vi "ScanXY.vi"(11 "Scan/Meas Parameters":T1={"Pixel Dwell Time (s)"=0.0001, "Pixel Size"=200.0, "X Min (V)"=-7.5, "X Max (V)"=7.5, "Y Min (V)"=-7.5, "Y Max (V)"=7.5, "XY Factor (1/V)"=0.2}) -> (3 "XYcoordinates":dbl[][](array[numeric]))   [LabVIEW 2018]
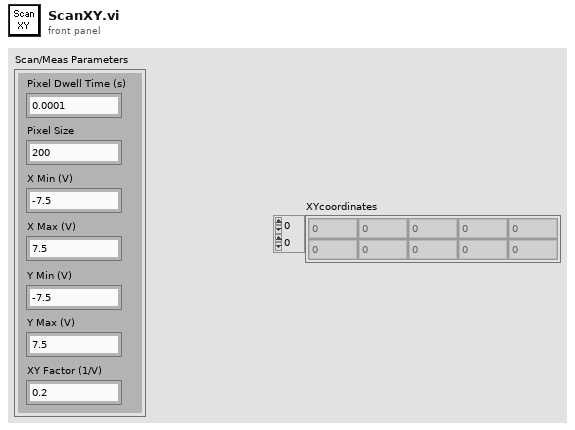
[diagram p1: front panel]
types:
  T1 = cluster{"Pixel Dwell Time (s)":dbl, "Pixel Size":dbl, "X Min (V)":dbl, "X Max (V)":dbl, "Y Min (V)":dbl, "Y Max (V)":dbl, "XY Factor (1/V)":dbl}
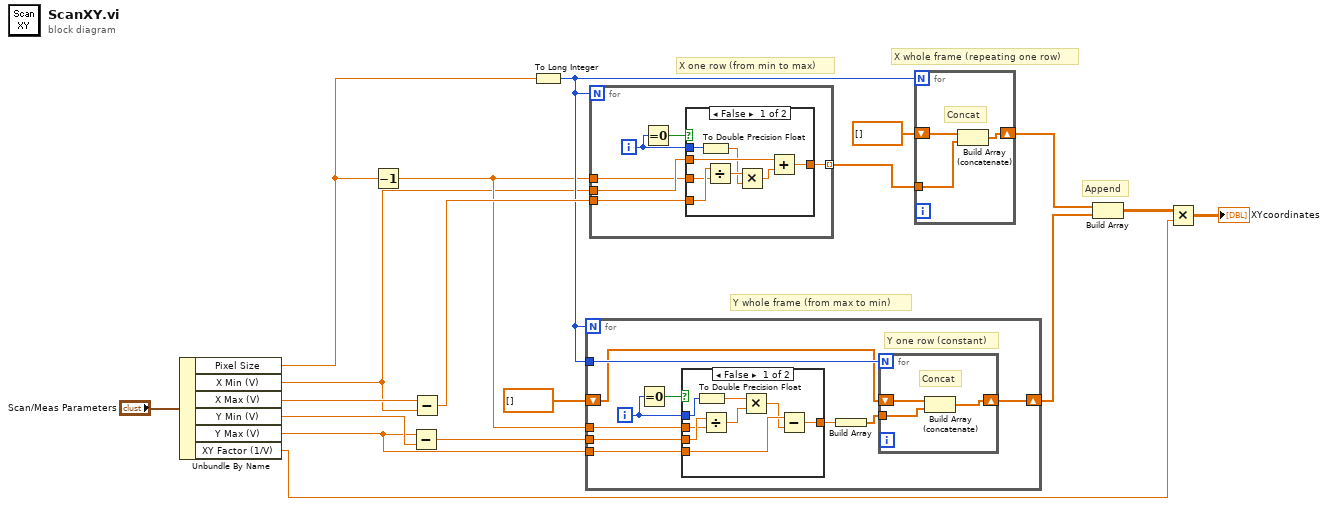
[diagram p0: block diagram]
diagram:
  # "Append"
  # "Y whole frame (from max to min)"
  # "X whole frame (repeating one row)"
  # "X one row (from min to max)"
  n1 = Unbundle By Name("Scan/Meas Parameters") -> ("Pixel Size"=w7:dbl, "X Min (V)"=w5:dbl, "X Max (V)"=w6:dbl, "Y Min (V)"=w4:dbl, "Y Max (V)"=w3:dbl, "XY Factor (1/V)"=w2:dbl)
  n2 = Decrement(x=w7) -> (x-1=w9:dbl)
  n3 = Subtract(x=w3, y=w4) -> (x-y=w14:dbl)
  n4 = Subtract(x=w6, y=w5) -> (x-y=w17:dbl)
  n5 = To Long Integer(number=w7) -> (32bit integer=w10:i32)
  n6 = for {
    N: w10 -> [_]
    tunnel: w3 -> [w27]
    tunnel: w14 -> [w26]
    tunnel: w9 -> [w25]
    tunnel: w10 -> [w22]
    shift-right: [w20] -> w11
    shift-left: dbl[] [] -> [w19]
    i -> [w24]
    # "Y one row (constant)"
    n7 = Equal To 0?(x=w24) -> (x = 0?=w28:bool)
    n8 = case shown="False" w28 {
      tunnel: w27 -> [w39 w40]
      tunnel: [w35 w40] -> w23
      tunnel: w26 -> [w38 _]
      tunnel: w25 -> [w37 _]
      tunnel: w24 -> [w33 _]
      frame False {
        n9 = To Double Precision Float(number=w33) -> (double precision float=w32:dbl)
        n10 = Divide(x=w38, y=w37) -> (x/y=w34:dbl)
        n11 = Multiply(x=w32, y=w34) -> (x*y=w36:dbl)
        n12 = Subtract(x=w39, y=w36) -> (x-y=w35:dbl)
      }
      frame True {
      }
    }
    n13 = Build Array(w23) -> (w21:dbl[])
    n14 = for {
      N: w22 -> [_]
      shift-right: [w29] -> w20
      shift-left: w19 -> [w31]
      tunnel: w21 -> [w30]
      # "Concat"
      n15 = Build Array (concatenate)(w31, w30) -> (w29:dbl[])
    }
  }
  n16 = for {
    N: w10 -> [_]
    tunnel: w5 -> [w44]
    tunnel: [w45] -> w16 mode=indexing
    tunnel: w17 -> [w43]
    tunnel: w9 -> [w42]
    i -> [w41]
    n17 = Equal To 0?(x=w41) -> (x = 0?=w46:bool)
    n18 = case shown="False" w46 {
      tunnel: w44 -> [w54 w55]
      tunnel: [w49 w55] -> w45
      tunnel: w43 -> [w53 _]
      tunnel: w42 -> [w52 _]
      tunnel: w41 -> [w48 _]
      frame False {
        n19 = To Double Precision Float(number=w48) -> (double precision float=w47:dbl)
        n20 = Divide(x=w53, y=w52) -> (x/y=w51:dbl)
        n21 = Multiply(x=w51, y=w47) -> (x*y=w50:dbl)
        n22 = Add(x=w54, y=w50) -> (x+y=w49:dbl)
      }
      frame True {
      }
    }
  }
  n23 = for {
    N: w10 -> [_]
    shift-right: [w57] -> w12
    shift-left: dbl[] [] -> [w58]
    tunnel: w16 -> [w56]
    # "Concat"
    n24 = Build Array (concatenate)(w58, w56) -> (w57:dbl[])
  }
  n25 = Build Array(w12, w11) -> (w8:dbl[][])
  n26 = Multiply(x=w8, y=w2) -> (x*y=→"XYcoordinates":dbl[][])
